vi "Destoyer UserEevents.vi"(8 "error in (no error)":errorcluster, 11 "Limites Contador in":refnum<class "Limites Contador.lvclass">) -> (0 "error out":errorcluster, 3 "Limites Contador out":refnum<class "Limites Contador.lvclass">)   [LabVIEW 2020, in "Limites Contador.lvlib" / "Limites Contador.lvclass"]
uses:
  Limites Contador.lvclass
  Limites Contador.lvclass/Limites Contador.ctl
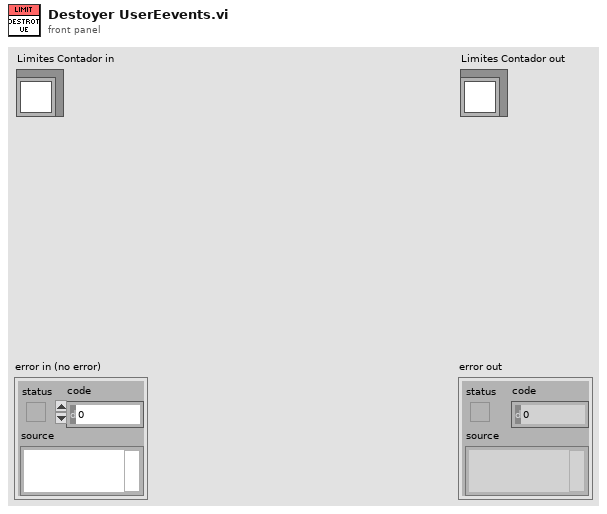
[diagram p1: front panel]
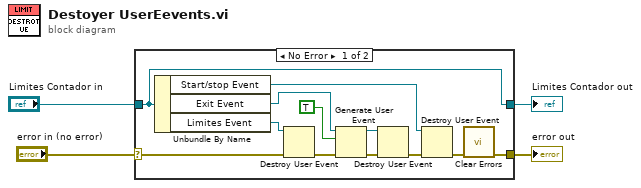
[diagram p0: block diagram]
diagram:
  n1 = case shown="No Error" "error in (no error)" {
    selector: "error in (no error)" -> [w9 w18]
    tunnel: [w10 w18] -> w3
    tunnel: [w16 w17] -> w1
    tunnel: "Limites Contador in" -> [w16 w17]
    frame No Error {
      n2 = Unbundle By Name(w16) -> ("Start/stop Event"=w15:refnum<user-event>, "Exit Event"=w14:refnum<user-event>, "Limites Event"=w11:refnum<user-event>)
      n3 = Destroy User Event(user event=w11, error in=w9) -> (error out=w8:errorcluster)
      n4 = Generate User Event(user event=w14, event data cluster=TRUE ("event data"), error in=w8) -> (user event out=w12:refnum<user-event>, error out=w7:errorcluster)  [unwired: 1 in]
      n5 = Destroy User Event(user event=w12, error in=w7) -> (error out=w6:errorcluster)
      n6 = Destroy User Event(user event=w15, error in=w6) -> (error out=w5:errorcluster)
      n7 = call <vilib>:"Clear Errors.vi"("error in (no error)"=w5) -> ("error out"=w10:errorcluster)  [unwired: 5 in, 1 out]
    }
    frame Error {
    }
  }
  "error out" <- w3
  "Limites Contador out" <- w1
